vi "IR_OPO_esp_gpib_comm_ASCII.vi"(3 "error in":errorcluster, 4 "Query?":bool=TRUE, 5 "Command":string="tb", 6 "GPIB Params":T1={"Port In"=1, "Delay"=0, "Timeout"=300, "TermChar"=0}) -> (0 "error out":errorcluster, 1 "Tmout?":bool, 2 "Response":string="0, 9622160, NO ERROR DETECTED\r\n")   [LabVIEW 2015]
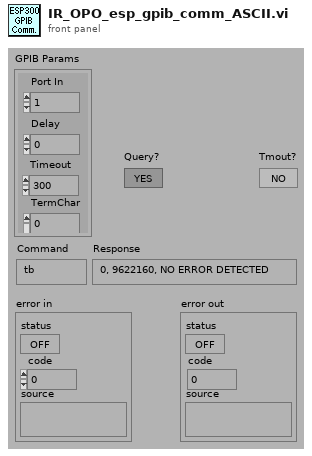
[diagram p1: front panel]
types:
  T1 = cluster{"Port In":i32, "Delay":u16, "Timeout":u16, "TermChar":u16}
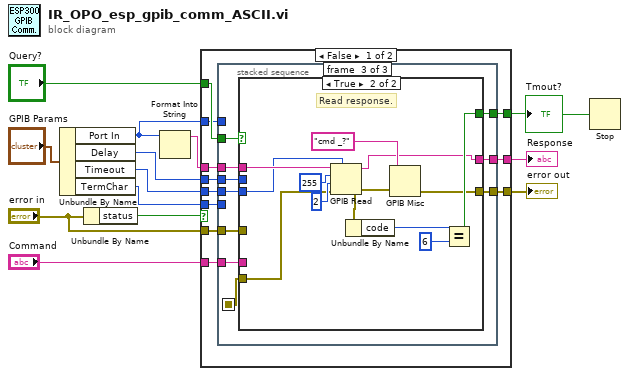
[diagram p0: block diagram]
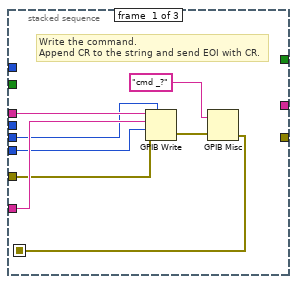
[diagram p2: hidden frame]
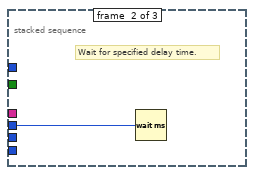
[diagram p3: hidden frame]
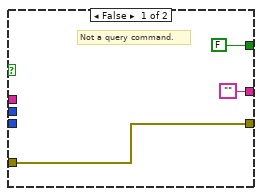
[diagram p4: hidden frame]
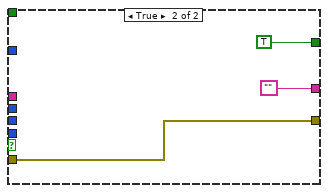
[diagram p5: hidden frame]
diagram:
  n1 = Unbundle By Name("GPIB Params") -> ("Port In"=w3:i32, "Delay"=w6:u16, "Timeout"=w5:u16, "TermChar"=w1:u16)
  n2 = Unbundle By Name("error in") -> ("status"=w10:bool)
  n3 = Format Into String(w3) -> (resulting string=w11:string)  [unwired: 3 in, 1 out]
  n4 = case shown="False" w10 {
    tunnel: "Command" -> [w24 _]
    tunnel: [w17 ""] -> w12
    tunnel: w11 -> [w23 _]
    tunnel: "error in" -> [w21 w60]
    tunnel: [w18 w60] -> w8
    tunnel: w6 -> [w22 _]
    tunnel: w5 -> [w20 _]
    tunnel: "Query?" -> [w19 _]
    tunnel: [w16 TRUE] -> w2
    tunnel: w3 -> [w15 _]
    tunnel: w1 -> [w14 _]
    frame False {
      n5 = stacked-sequence {
        seq-local: [w25 _ _] -> [_ _ w35]
        tunnel: w24 -> [w31 _ w34]
        tunnel: w23 -> [w32 _ w43]
        tunnel: w22 -> [_ w33 w39]
        tunnel: w21 -> [w30 _ w37]
        tunnel: w20 -> [w28 _ w40]
        tunnel: w19 -> [_ _ w42]
        tunnel: [_ _ w41] -> w18
        tunnel: [_ _ w38] -> w17
        tunnel: [_ _ w36] -> w16
        tunnel: w15 -> [_ _ _]
        tunnel: w14 -> [w29 _ _]
        frame #0 {
          # "Write the command.\nAppend CR to the string and send EOI with CR."
          n6 = GPIB Write(0:w32, 1:w31, 2:w29, 3:w30, 4:w28) -> (6:w27:errorcluster)  [unwired: 1 out]
          n7 = GPIB Misc(0:"cmd _?" ("command string"), 1:w27) -> (4:w25:errorcluster)  [unwired: 2 out]
        }
        frame #1 {
          # "Wait for specified delay time."
          n8 = Wait (ms)(milliseconds to wait=w33) -> ()  [unwired: 1 out]
        }
        frame #2 {
          n9 = case shown="True" w42 {
            tunnel: w43 -> [_ w58]
            tunnel: [w45 w47] -> w41
            tunnel: w40 -> [_ w53]
            tunnel: w39 -> [_ _]
            tunnel: ["" w49] -> w38
            tunnel: w37 -> [w45 _]
            tunnel: [FALSE w51] -> w36
            tunnel: w35 -> [_ w54]
            tunnel: w34 -> [_ _]
            frame False {
              # "Not a query command."
            }
            frame True {
              # "Read response."
              n10 = GPIB Read(0:w58, 1:255 ("byte count"), 2:i16 2 ("mode (0)"), 3:w54, 4:w53) -> (5:w49:string, 7:w48:errorcluster)  [unwired: 1 out]
              n11 = Unbundle By Name(w48) -> ("code"=w50:i32)
              n12 = GPIB Misc(0:"cmd _?" ("command string"), 1:w48) -> (4:w47:errorcluster)  [unwired: 2 out]
              n13 = Equal?(x=w50, y=6) -> (x = y?=w51:bool)
            }
          }
        }
      }
    }
    frame True {
    }
  }
  "Response" <- w12
  "error out" <- w8
  "Tmout?" <- w2
  n14 = Stop(stop? (T)=w2) -> ()
